vi "AudioTest.Adjust Floating Limits.vi"(7 "Lim Name":string, 10 "LimitPlots":T1[](array[typedef]), 11 "Plot":T1) -> (2 "LimitPlots Out":T1[](array[typedef]))   [LabVIEW 2018]
uses:
  TypeDefs/AudioTest.Result Plot Data.ctl
panel:
  out "XY Graph":cluster{"X":dbl[], "Y":dbl[]}[](graph)
  out "Adj":dbl
  out "LL Margin":dbl
  out "UL Margin":dbl
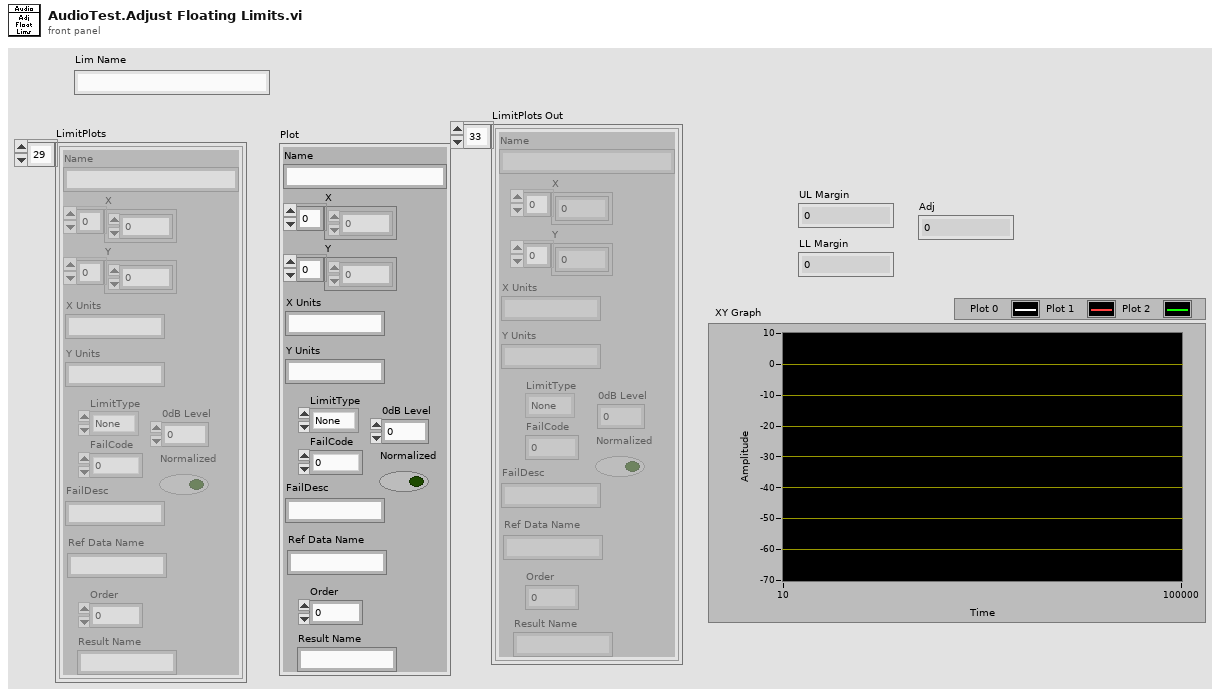
[diagram p1: front panel]
types:
  T1 = typedef "AudioTest.Result Plot Data.ctl" = cluster{"Order":i32, "Name":string, "X":dbl[], "Y":dbl[], "X Units":string, "Y Units":string, "LimitType":enum16{"None", "LL", "UL"}, "FailCode":i32, "FailDesc":string, "Ref Data Name":string, "Result Name":string, "0dB Level":dbl, "Normalized":bool}
  T2 = cluster{"UL":T1, "LL":T1, "Plot":T1, "iUL":i32, "iLL":i32, "Side":string}
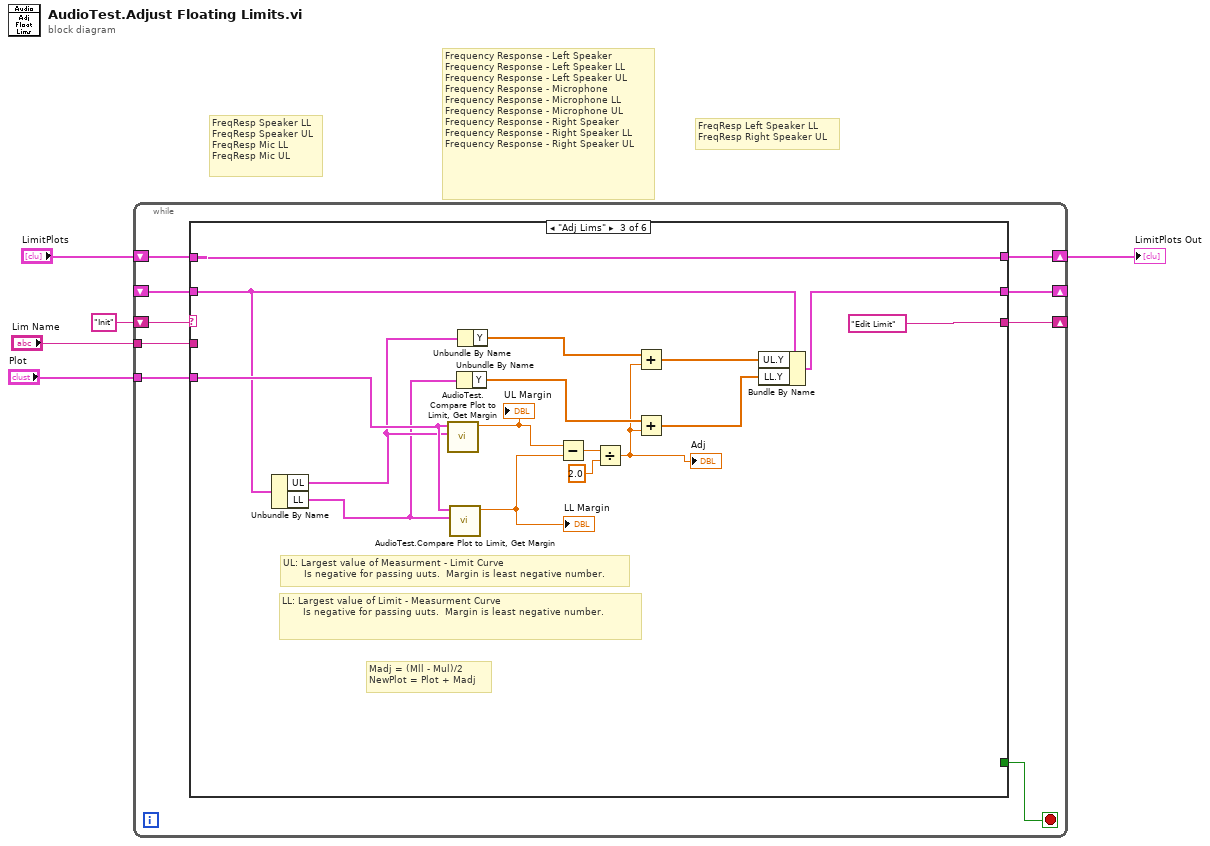
[diagram p0: block diagram]
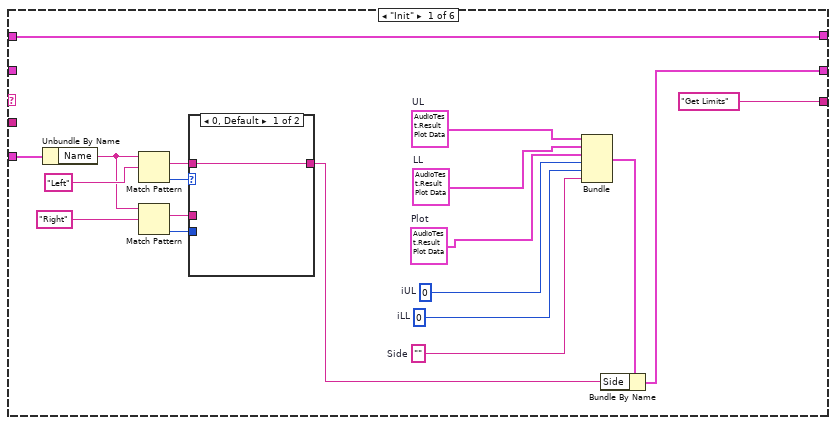
[diagram p2: hidden frame]
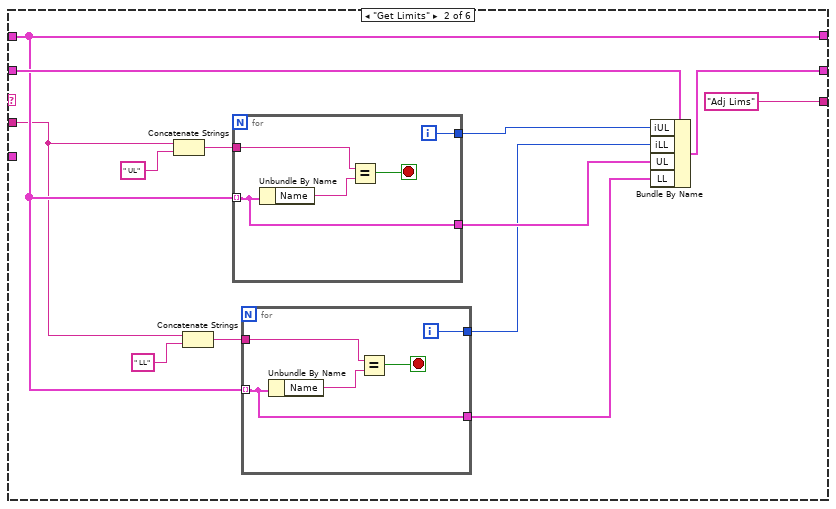
[diagram p5: hidden frame]
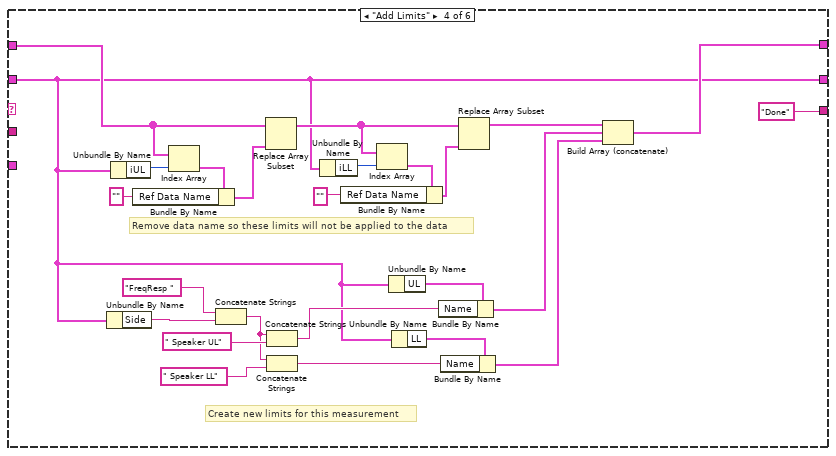
[diagram p6: hidden frame]
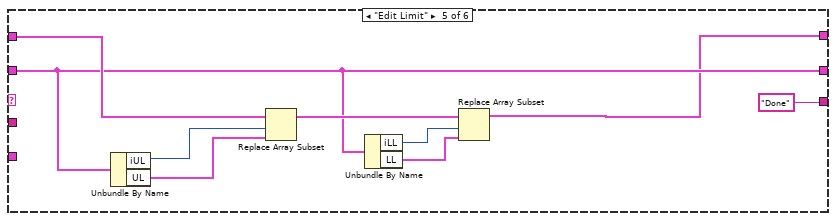
[diagram p7: hidden frame]
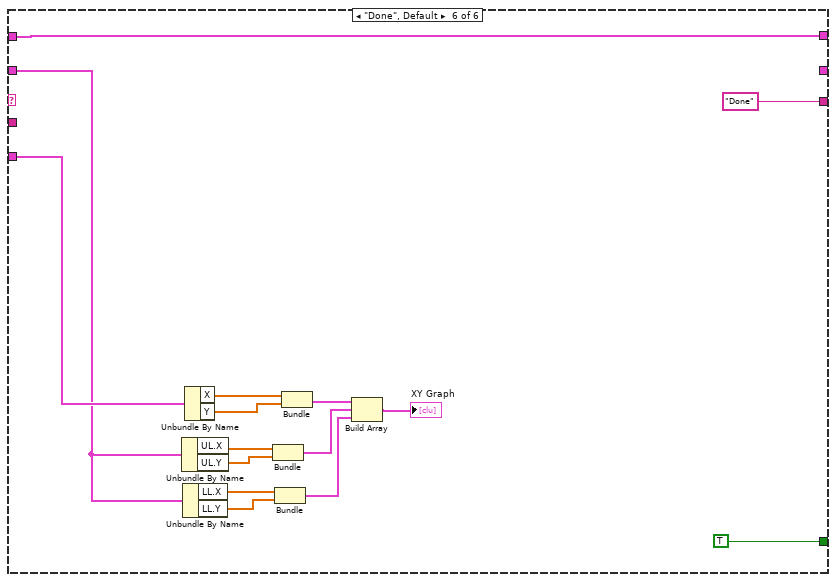
[diagram p8: hidden frame]
diagram:
  # "FreqResp Left Speaker LL\nFreqResp Right Speaker UL"
  # "FreqResp Speaker LL\nFreqResp Speaker UL\nFreqResp Mic LL\nFreqResp Mic UL"
  # "Frequency Response - Left Speaker\nFrequency Response - Left Speaker LL\nFrequency Response - Left Speaker UL\nFrequency Response - Microphone\nFrequency Response - Microphone LL\nFrequency Response - Microphone UL\nFrequency Response - Right Speaker\nFrequency Response - Right Speaker LL\nFrequency Response - Right Speaker UL"
  n1 = while {
    tunnel: "Plot" -> [w14]
    shift-right: [w11] -> _
    shift-left: _ -> [w9]
    shift-right: [w8] -> _
    shift-left: "Init" -> [w12]
    tunnel: "Lim Name" -> [w6]
    shift-right: [w7] -> w2
    shift-left: "LimitPlots" -> [w13]
    stop <- w10 stop-if-true
    n2 = case shown="\"Adj Lims\"" w12 {
      tunnel: w14 -> [w27 _ w77 _ _ w114]
      tunnel: w13 -> [w16 w44 w63 w90 w111 w112]
      tunnel: [w23 w50 w64 w80 w109 _] -> w11
      tunnel: [_ _ _ _ _ TRUE] -> w10
      tunnel: w9 -> [_ w51 w73 w80 w109 w113]
      tunnel: ["Get Limits" "Adj Lims" "Edit Limit" "Done" "Done" "Done"] -> w8
      tunnel: [w16 w44 w63 w92 w107 w112] -> w7
      tunnel: w6 -> [_ w39 _ _ _ _]
      frame "Init" {
        w25 = ""  # Side
        w29 = 0  # iUL
        w28 = 0  # iLL
        w30 = T1 {"Order"=0, "Name"="", "X"=[], "Y"=[], "X Units"="", "Y Units"="", "LimitType"=enum."None", "FailCode"=0, "FailDesc"="", "Ref Data Name"="", "Result Name"="", "0dB Level"=0.0, "Normalized"=FALSE}  # Plot
        w33 = T1 {"Order"=0, "Name"="", "X"=[], "Y"=[], "X Units"="", "Y Units"="", "LimitType"=enum."None", "FailCode"=0, "FailDesc"="", "Ref Data Name"="", "Result Name"="", "0dB Level"=0.0, "Normalized"=FALSE}  # UL
        w32 = T1 {"Order"=0, "Name"="", "X"=[], "Y"=[], "X Units"="", "Y Units"="", "LimitType"=enum."None", "FailCode"=0, "FailDesc"="", "Ref Data Name"="", "Result Name"="", "0dB Level"=0.0, "Normalized"=FALSE}  # LL
        n3 = Unbundle By Name(w27) -> ("Name"=w15:string)
        n4 = Match Pattern(string=w15, regular expression="Left") -> (match substring=w20:string, offset past match=w21:i32)  [unwired: 1 in, 2 out]
        n5 = Match Pattern(string=w15, regular expression="Right") -> (match substring=w19:string, offset past match=w18:i32)  [unwired: 1 in, 2 out]
        n6 = case shown="0, Default" w21 {
          tunnel: w20 -> [w34 _]
          tunnel: w19 -> [_ w35]
          tunnel: w18 -> [_ w37]
          tunnel: [w34 w36] -> w17
          frame 0, Default {
          }
          frame -1 {
            n7 = case shown="0, Default" w37 {
              tunnel: [w38 _] -> w36
              tunnel: w35 -> [w38 _]
              frame 0, Default {
              }
              frame -1 {
              }
            }
          }
        }
        n8 = Bundle("UL"=w33, "LL"=w32, "Plot"=w30, "iUL"=w29, "iLL"=w28, "Side"=w25) -> (w24:T2)  [unwired: 1 in]
        n9 = Bundle By Name(cluster=w24, "Side"=w17) -> (w23:T2)
      }
      frame "Get Limits" {
        n10 = Concatenate Strings(w39, " UL" ("string")) -> (w48:string)
        n11 = Concatenate Strings(w39, " LL" ("string")) -> (w46:string)
        n12 = for {
          tunnel: w48 -> [w61]
          tunnel: w44 -> [w59] mode=indexing
          tunnel: [w59] -> w47
          tunnel: [w57] -> w41
          i -> [w57]
          stop <- w58 stop-if-true
          n13 = Unbundle By Name(w59) -> ("Name"=w60:string)
          n14 = Equal?(x=w61, y=w60) -> (x = y?=w58:bool)
        }
        n15 = for {
          tunnel: w46 -> [w56]
          tunnel: w44 -> [w54] mode=indexing
          tunnel: [w54] -> w43
          tunnel: [w52] -> w40
          i -> [w52]
          stop <- w53 stop-if-true
          n16 = Unbundle By Name(w54) -> ("Name"=w55:string)
          n17 = Equal?(x=w56, y=w55) -> (x = y?=w53:bool)
        }
        n18 = Bundle By Name(cluster=w51, "iUL"=w41, "iLL"=w40, "UL"=w47, "LL"=w43) -> (w50:T2)
      }
      frame "Adj Lims" {
        # "Madj = (Mll - Mul)/2\nNewPlot = Plot + Madj"
        # "LL: Largest value of Limit - Measurment Curve\n       Is negative for passing uuts.  Margin is least negative number."
        # "UL: Largest value of Measurment - Limit Curve\n       Is negative for passing uuts.  Margin is least negative number."
        n19 = Unbundle By Name(w73) -> ("UL"=w70:T1, "LL"=w69:T1)
        n20 = call "AudioTest.Compare Plot to Limit, Get Margin.vi"("Plot Limit"=w70, "Plot Data"=w77) -> ("Margin"=w74:dbl)  [unwired: 8 in, 1 out]
        "UL Margin" <- w74
        n21 = call "AudioTest.Compare Plot to Limit, Get Margin.vi"("Plot Limit"=w69, "Plot Data"=w77) -> ("Margin"=w66:dbl)  [unwired: 8 in, 1 out]
        "LL Margin" <- w66
        n22 = Unbundle By Name(w69) -> ("Y"=w68:dbl[])
        n23 = Unbundle By Name(w70) -> ("Y"=w67:dbl[])
        n24 = Subtract(x=w74, y=w66) -> (x-y=w76:dbl)
        n25 = Divide(x=w76, y=2.0) -> (x/y=w65:dbl)
        "Adj" <- w65
        n26 = Add(x=w67, y=w65) -> (x+y=w72:dbl[])
        n27 = Add(x=w68, y=w65) -> (x+y=w71:dbl[])
        n28 = Bundle By Name(cluster=w73, "UL.Y"=w72, "LL.Y"=w71) -> (w64:T2)
      }
      frame "Add Limits" {
        # "Create new limits for this measurement"
        # "Remove data name so these limits will not be applied to the data"
        n29 = Unbundle By Name(w80) -> ("Side"=w91:string)
        n30 = Unbundle By Name(w80) -> ("iUL"=w89:i32)
        n31 = Index Array(array=w90, index=w89) -> (element=w88:T1)
        n32 = Bundle By Name(cluster=w88, "Ref Data Name"="") -> (w86:T1)
        n33 = Concatenate Strings("FreqResp " ("regular expression"), w91) -> (w99:string)
        n34 = Replace Array Subset(array=w90, new element=w86) -> (w81:T1[])  [unwired: 1 in]
        n35 = Concatenate Strings(w99, " Speaker UL" ("string")) -> (w97:string)
        n36 = Concatenate Strings(w99, " Speaker LL" ("string")) -> (w95:string)
        n37 = Unbundle By Name(w80) -> ("iLL"=w85:i32)
        n38 = Index Array(array=w81, index=w85) -> (element=w84:T1)
        n39 = Bundle By Name(cluster=w84, "Ref Data Name"="") -> (w82:T1)
        n40 = Unbundle By Name(w80) -> ("UL"=w98:T1)
        n41 = Unbundle By Name(w80) -> ("LL"=w94:T1)
        n42 = Bundle By Name(cluster=w98, "Name"=w97) -> (w96:T1)
        n43 = Bundle By Name(cluster=w94, "Name"=w95) -> (w93:T1)
        n44 = Replace Array Subset(array=w81, new element=w82) -> (w79:T1[])  [unwired: 1 in]
        n45 = Build Array (concatenate)(w79, w96, w93) -> (w92:T1[])
      }
      frame "Edit Limit" {
        n46 = Unbundle By Name(w109) -> ("iUL"=w106:i32, "UL"=w105:T1)
        n47 = Replace Array Subset(array=w111, new element=w105, index=w106) -> (w110:T1[])
        n48 = Unbundle By Name(w109) -> ("iLL"=w104:i32, "LL"=w103:T1)
        n49 = Replace Array Subset(array=w110, new element=w103, index=w104) -> (w107:T1[])
      }
      frame "Done", Default {
        n50 = Unbundle By Name(w113) -> ("UL.X"=w122:dbl[], "UL.Y"=w121:dbl[])
        n51 = Unbundle By Name(w113) -> ("LL.X"=w124:dbl[], "LL.Y"=w123:dbl[])
        n52 = Unbundle By Name(w114) -> ("X"=w120:dbl[], "Y"=w119:dbl[])
        n53 = Bundle("X"=w122, "Y"=w121) -> (w117:cluster{"X":dbl[], "Y":dbl[]})  [unwired: 1 in]
        n54 = Bundle("X"=w124, "Y"=w123) -> (w116:cluster{"X":dbl[], "Y":dbl[]})  [unwired: 1 in]
        n55 = Bundle("X"=w120, "Y"=w119) -> (w118:cluster{"X":dbl[], "Y":dbl[]})  [unwired: 1 in]
        n56 = Build Array(w118, w117, w116) -> (→"XY Graph":cluster{"X":dbl[], "Y":dbl[]}[])
      }
    }
  }
  "LimitPlots Out" <- w2
